vi "Light.vi"(8 "错误常量":errorcluster, 11 "IO Name":string[](array[string])=["Green", "Yellow", "Red", "Buzzing"]) -> (0 "error out":errorcluster)   [LabVIEW 2017]
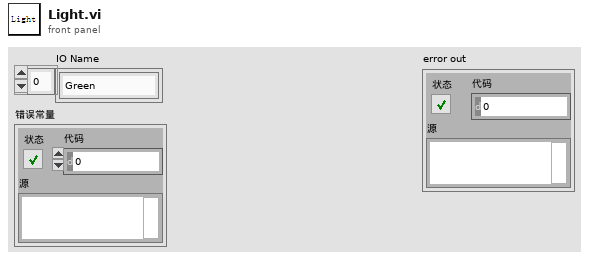
[diagram p1: front panel]
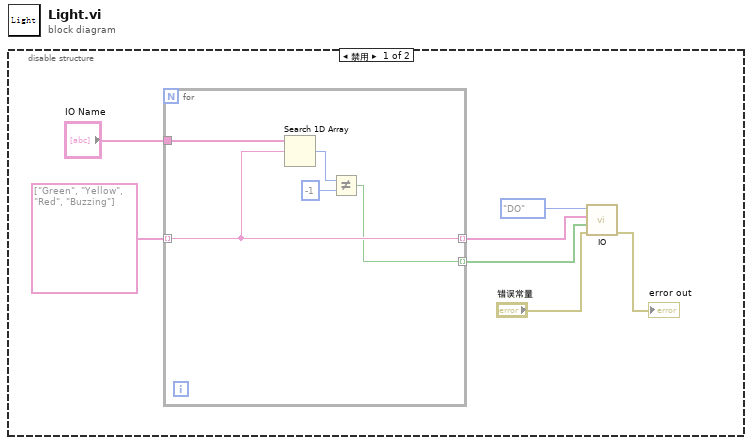
[diagram p0: block diagram]
diagram:
  n1 = disable-structure shown="禁用" {
    frame Disabled {
      n2 = for {
        tunnel: string[] ["Green", "Yellow", "Red", "Buzzing"] ("IO Name") -> [w9] mode=indexing
        tunnel: "IO Name" -> [w12]
        tunnel: [w9] -> w4 mode=indexing
        tunnel: [w8] -> w3 mode=indexing
        n3 = Search 1D Array(1D array=w12, element=w9) -> (index of element=w11:i32)  [unwired: 1 in]
        n4 = Not Equal?(x=w11, y=-1) -> (x != y?=w8:bool)
      }
      n5 = call "IO.vi"("错误常量"="错误常量", "DO DATA"=w3, "IO Name"=w4, "IO?"=enum16{"DI", "DO"}."DO") -> ("error out"=→"error out":errorcluster)  [unwired: 6 in, 1 out]
    }
    frame Enabled {
    }
  }
